vi "save configuration.vi"(8 "error in (no error)":errorcluster, 10 "filename":string, 11 "path":path) -> (0 "error out":errorcluster)   [LabVIEW 2015]
uses:
  global variables/params.vi
  <vilib>/Utility/config.llb/Write Key (String).vi
  <vilib>/Utility/config.llb/NI_LVConfig.lvlib
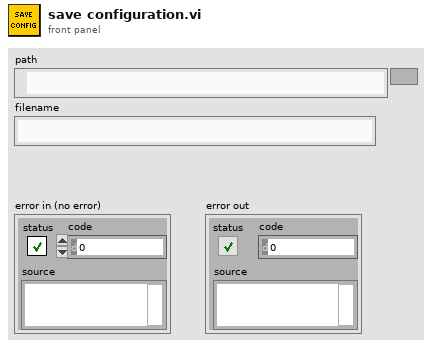
[diagram p1: front panel]
types:
  T1 = typedef "NI_LVConfig.lvlib/Config Data RefNum.ctl" = refnum<k1>
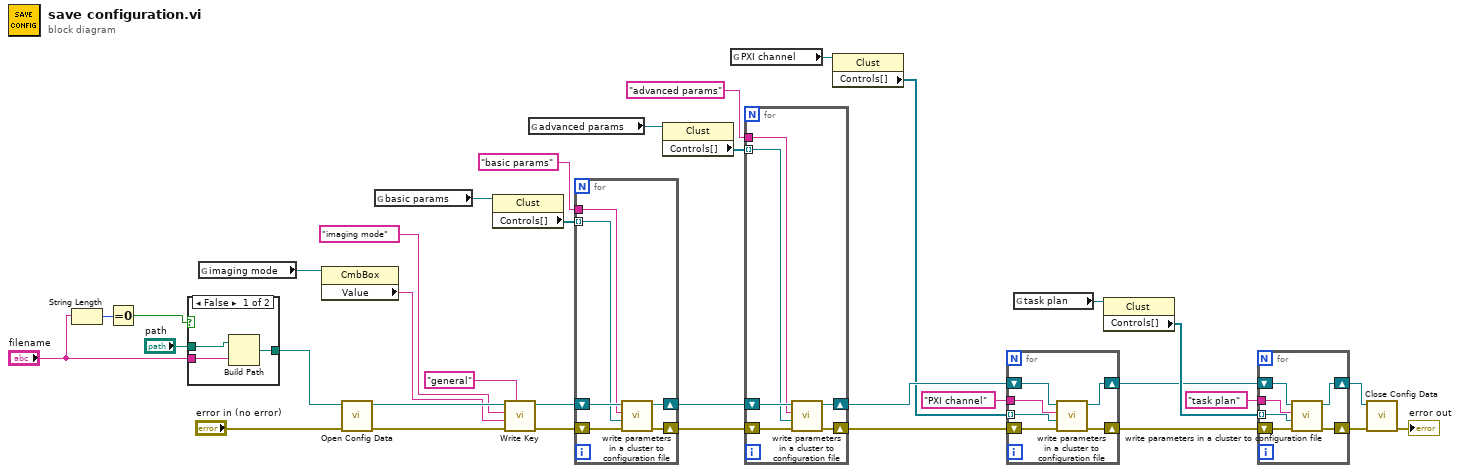
[diagram p0: block diagram]
diagram:
  n1 = String Length(string="filename") -> (length=w5:i32)
  n2 = Equal To 0?(x=w5) -> (x = 0?=w4:bool)
  n3 = case shown="False" w4 {
    tunnel: "filename" -> [w37 _]
    tunnel: [w38 w39] -> w3
    tunnel: "path" -> [w36 w39]
    frame False {
      n4 = Build Path(base path=w36, name or relative path=w37) -> (appended path=w38:path)
    }
    frame True {
    }
  }
  n5 = global read "params.vi" "imaging mode"() -> (w20:refnum<vi>)
  n6 = property class="CmbBox"(reference=w20) -> ("Value"=w23:string)  [unwired: 1 in, 2 out]
  n7 = call <vilib>:"Open Config Data.vi"("error in (no error)"="error in (no error)", "configuration file path"=w3) -> ("error out"=w28:errorcluster, "refnum"=w30:T1)  [unwired: 7 in, 1 out]
  n8 = global read "params.vi" "basic params"() -> (w14:refnum<vi>)
  n9 = property class="Clust"(reference=w14) -> ("Controls[]"=w22:refnum<vi>[])  [unwired: 1 in, 2 out]
  n10 = call-poly <vilib>:"Write Key.vi"("section"="general", "error in (no error)"=w28, "value"=w23, "key"="imaging mode", "refnum"=w30) -> ("error out"=w29:errorcluster, "refnum out"=w31:T1)  [unwired: 4 in, 1 out]
  n11 = global read "params.vi" "advanced params"() -> (w19:refnum<vi>)
  n12 = for {
    tunnel: "basic params" -> [w44]
    tunnel: w22 -> [w42] mode=indexing
    shift-right: [w41] -> w24
    shift-left: w31 -> [w45]
    shift-right: [w40] -> w25
    shift-left: w29 -> [w43]
    n13 = call "write parameters in a cluster to configuration file.vi"("error in (no error)"=w43, "Control in"=w42, "section"=w44, "refnum"=w45) -> ("error out"=w40:errorcluster, "refnum out"=w41:T1)  [unwired: 4 in]
  }
  n14 = property class="Clust"(reference=w19) -> ("Controls[]"=w21:refnum<vi>[])  [unwired: 1 in, 2 out]
  n15 = global read "params.vi" "PXI channel"() -> (w15:refnum<vi>)
  n16 = for {
    tunnel: "advanced params" -> [w50]
    tunnel: w21 -> [w48] mode=indexing
    shift-right: [w47] -> w17
    shift-left: w24 -> [w51]
    shift-right: [w46] -> w16
    shift-left: w25 -> [w49]
    n17 = call "write parameters in a cluster to configuration file.vi"("error in (no error)"=w49, "Control in"=w48, "section"=w50, "refnum"=w51) -> ("error out"=w46:errorcluster, "refnum out"=w47:T1)  [unwired: 4 in]
  }
  n18 = property class="Clust"(reference=w15) -> ("Controls[]"=w13:refnum<vi>[])  [unwired: 1 in, 2 out]
  n19 = for {
    tunnel: "PXI channel" -> [w56]
    tunnel: w13 -> [w54] mode=indexing
    shift-right: [w53] -> w9
    shift-left: w17 -> [w57]
    shift-right: [w52] -> w6
    shift-left: w16 -> [w55]
    n20 = call "write parameters in a cluster to configuration file.vi"("error in (no error)"=w55, "Control in"=w54, "section"=w56, "refnum"=w57) -> ("error out"=w52:errorcluster, "refnum out"=w53:T1)  [unwired: 4 in]
  }
  n21 = global read "params.vi" "task plan"() -> (w12:refnum<vi>)
  n22 = property class="Clust"(reference=w12) -> ("Controls[]"=w11:refnum<vi>[])  [unwired: 1 in, 2 out]
  n23 = for {
    tunnel: w11 -> [w63] mode=indexing
    tunnel: "task plan" -> [w62]
    shift-right: [w59] -> w7
    shift-left: w6 -> [w58]
    shift-right: [w60] -> w8
    shift-left: w9 -> [w61]
    n24 = call "write parameters in a cluster to configuration file.vi"("error in (no error)"=w58, "Control in"=w63, "section"=w62, "refnum"=w61) -> ("error out"=w59:errorcluster, "refnum out"=w60:T1)  [unwired: 4 in]
  }
  n25 = call <vilib>:"Close Config Data.vi"("error in (no error)"=w7, "refnum"=w8) -> ("error out"=→"error out":errorcluster)  [unwired: 8 in, 1 out]
